vi "Initialize Unique String Buffer.vi"() -> (0 "Buffer out":refnum<class "Unique String Buffer.lvclass">)   [LabVIEW 2015, in "SLSC Switch.lvlib" / "Unique String Buffer.lvclass"]
uses:
  Unique String Buffer.lvclass
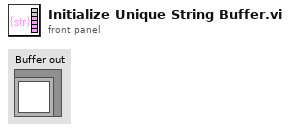
[diagram p1: front panel]
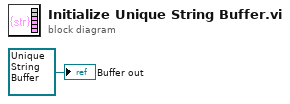
[diagram p0: block diagram]
diagram:
  "Buffer out" <- refnum<class "Unique String Buffer.lvclass"> refnum ("SLSC Switch.lvlib:Unique String Buffer.lvclass")
